vi "Select_inst_info.vi"(1 "Inst_parameters.Inst_array":T1(array[cluster]), 2 "Initial move":T2(array[cluster])) -> (0 "Inst_parameters.Inst_array 2":T1(array[cluster]))   [LabVIEW 2013]
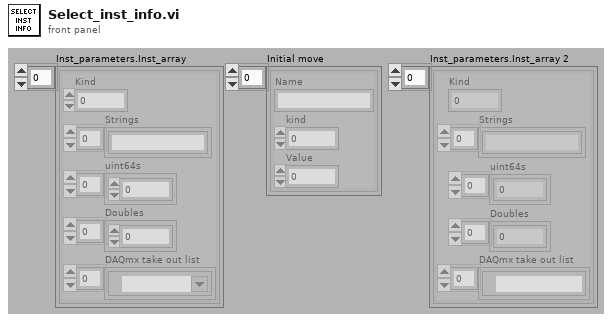
[diagram p1: front panel]
types:
  T1 = cluster{"Kind":u16, "Strings":string[], "uint64s":u64[], "Doubles":dbl[], "DAQmx take out list":refnum<k21>[]}[]
  T2 = cluster{"Name":string, "kind":u64, "Value":dbl}[]
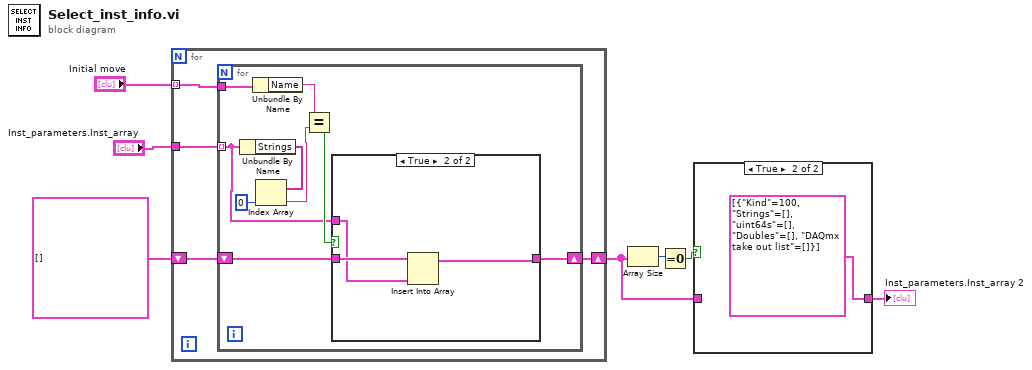
[diagram p0: block diagram]
diagram:
  n1 = for {
    tunnel: "Initial move" -> [w11] mode=indexing
    shift-right: [w8] -> w2
    shift-left: T1 [] ("Inst_parameters.Inst_array 2") -> [w9]
    tunnel: "Inst_parameters.Inst_array" -> [w10]
    n2 = for {
      tunnel: w11 -> [w20]
      tunnel: w10 -> [w12] mode=indexing
      shift-right: [w13] -> w8
      shift-left: w9 -> [w14]
      n3 = Unbundle By Name(w12) -> ("Strings"=w19:string[])
      n4 = Unbundle By Name(w20) -> ("Name"=w17:string)
      n5 = Index Array(array=w19, index=0) -> (element=w16:string)
      n6 = Equal?(x=w17, y=w16) -> (x = y?=w15:bool)
      n7 = case shown="True" w15 {
        tunnel: w14 -> [w21 w24]
        tunnel: [w21 w23] -> w13
        tunnel: w12 -> [_ w22]
        frame False {
        }
        frame True {
          n8 = Insert Into Array(array=w24, new element=w22) -> (w23:T1)  [unwired: 1 in]
        }
      }
    }
  }
  n9 = Array Size(array=w2) -> (size(s)=w4:i32)
  n10 = Equal To 0?(x=w4) -> (x = 0?=w3:bool)
  n11 = case shown="True" w3 {
    tunnel: w2 -> [w25 _]
    tunnel: [w25 T1 [{"Kind"=100, "Strings"=[], "uint64s"=[], "Doubles"=[], "DAQmx take out list"=[]}] ("Inst_parameters.Inst_array 2")] -> w1
    frame False {
    }
    frame True {
    }
  }
  "Inst_parameters.Inst_array 2" <- w1
